vi "Release Session.vi"(0 "Session Handle":T1, 11 "error in (no error)":errorcluster, 13 "force destroy? (F)":bool) -> (15 "error out":errorcluster)   [LabVIEW 2020, in "TSS.lvlib" / "VariableContainer.lvclass"]
doc: "Releases an obtained reference to the session"
uses:
  VariableContainer.lvclass
  Typedefs/Session Handle.ctl
  C:/Program Files (x86)/National Instruments/LabVIEW 2020/user.lib/_Session Fwk/Session - Root.lvclass
  Get Engine.vi
  Engine/Engine.lvclass
  <userlib>/_Session Fwk/Session - Root.lvclass
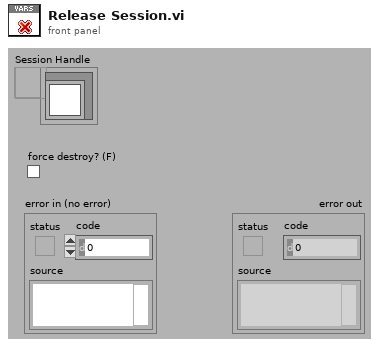
[diagram p1: front panel]
types:
  T1 = typedef "TSS.lvlib/VariableContainer.lvclass/Session Handle.ctl" = refnum<data-value>
  T2 = typedef "TSS.lvlib/Engine.lvclass/Session Handle.ctl" = refnum<data-value>
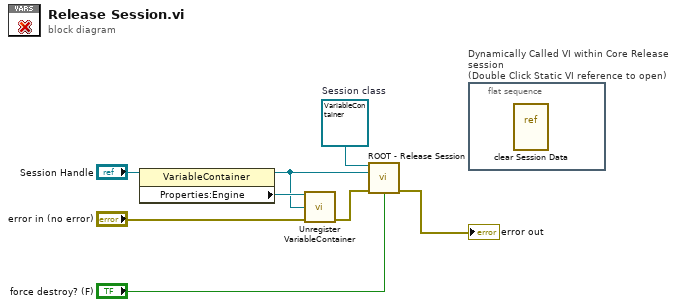
[diagram p0: block diagram]
diagram:
  w5 = refnum<class "VariableContainer.lvclass"> refnum  # Session class
  n1 = property class="VariableContainer"(reference="Session Handle") -> (reference out=w2:T1, "Properties:Engine"=w4:T2)  [unwired: 1 in, 1 out]
  n2 = call "Unregister VariableContainer.vi"("Session Handle in"=w4, "VariableContainer"=w2, "error in (no error)"="error in (no error)") -> ("error out"=w1:errorcluster)  [unwired: 11 in, 1 out]
  n3 = call <userlib>:"ROOT - Release Session.vi"("OBJ - Session in"=w5, "Session Handle in"=w2, "error in (no error)"=w1, "force destroy? (F)"="force destroy? (F)") -> ("error out"=→"error out":errorcluster)  [unwired: 10 in, 1 out]
  n4 = flat-sequence "Dynamically Called VI within Core Release session\n(Double Click Static VI reference to open)" {
    frame #0 {
      n5 = vi-ref "clear Session Data.vi"() -> ()  [unwired: 1 out]
    }
  }
